vi "Write wavelength2.vi"(8 "error in (no error)":errorcluster, 10 "wavelength2":dbl[unit]=6e-07 min=3e-07 max=9.999999999999999e-06, 11 "TCSAtmosphericDispersionStatus in":refnum<class "TCSAtmosphericDispersionStatus.lvclass">) -> (0 "error out":errorcluster, 3 "TCSAtmosphericDispersionStatus out":refnum<class "TCSAtmosphericDispersionStatus.lvclass">)   [LabVIEW 2014, in "TCSDataDefinitions.lvlib" / "TCSAtmosphericDispersionStatus.lvlib" / "TCSAtmosphericDispersionStatus.lvclass"]
uses:
  TCSAtmosphericDispersionStatus.lvclass
  TCSAtmosphericDispersionStatus.lvclass/TCSAtmosphericDispersionStatus.ctl
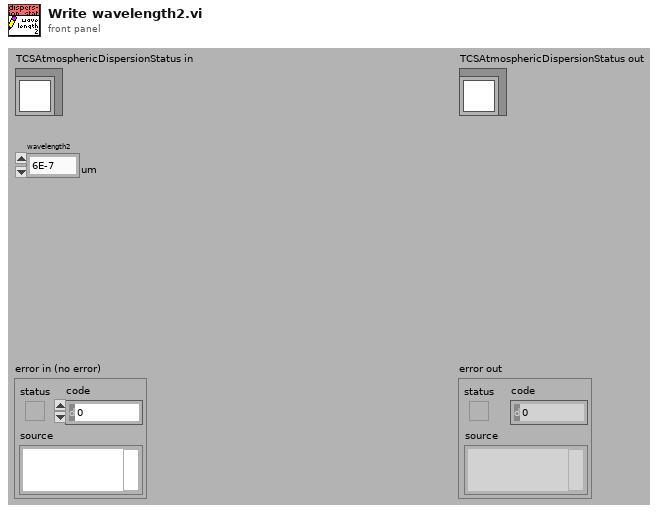
[diagram p1: front panel]
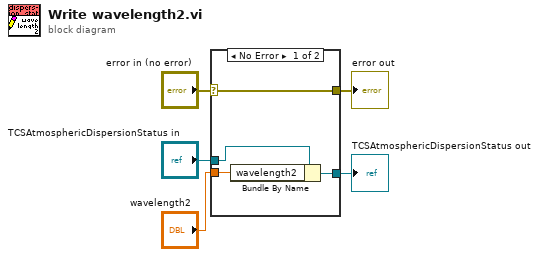
[diagram p0: block diagram]
diagram:
  n1 = case shown="No Error" "error in (no error)" {
    selector: "error in (no error)" -> [w9 w10]
    tunnel: [w9 w10] -> w4
    tunnel: [w7 w11] -> w2
    tunnel: "TCSAtmosphericDispersionStatus in" -> [w8 w11]
    tunnel: "wavelength2" -> [w6 _]
    frame No Error {
      n2 = Bundle By Name(cluster=w8, "wavelength2"=w6) -> (w7:refnum<class "TCSAtmosphericDispersionStatus.lvclass">)
    }
    frame Error {
    }
  }
  "error out" <- w4
  "TCSAtmosphericDispersionStatus out" <- w2
